vi "TargetUI.vi"() -> ()   [LabVIEW 2019, in "Target.lvclass"]
uses:
  Target.lvclass
  <vilib>/NI/Configuration Framework/Node/NodeRef.ctl
  <vilib>/NI/Configuration Framework/Node/NISE_CEF_Node.lvclass
  <vilib>/NI/AMC/Message Queue.ctl
  <vilib>/NI/AMC/Message.ctl
  <vilib>/NI/Tools/Keyed Array/KeyedArray.ctl
  <vilib>/NI/Configuration Framework/Node/UserEventRef.ctl
  <vilib>/NI/Configuration Framework/Controls/EventCluster.ctl
  C:/Program Files (x86)/National Instruments/LabVIEW 2019/vi.lib/NI/Configuration Framework/Node/NISE_CEF_Node.lvclass
  Target.lvclass/Target.ctl
  Read Source.vi
  Write Source.vi
  <vilib>/NI/AMC/Create Single Message.vi
  <vilib>/NI/AMC/Update Message Routing Info.vi
  <vilib>/NI/AMC/Send Message.vi
  <vilib>/NI/AMC/AMC.lvlib
  Configuration Tool.lvlib
  <vilib>/NI/Tools/Keyed Array/Tools_KeyedArray.lvlib
  <vilib>/NI/Configuration Framework/NISE_CEF_TreeControl.lvlib
panel:
  in  "Main UI Tab":enum32{"Target Information"}(tab)
  in  "Show Documentation":bool
  in  "Host Path to RT Driver VI":path
  in  "Real Time System Destination":string
  in  "user event":T1
  in  "main queue":T2
  in  "node ref":T3
  # "Host Information"
  # "Target Information"
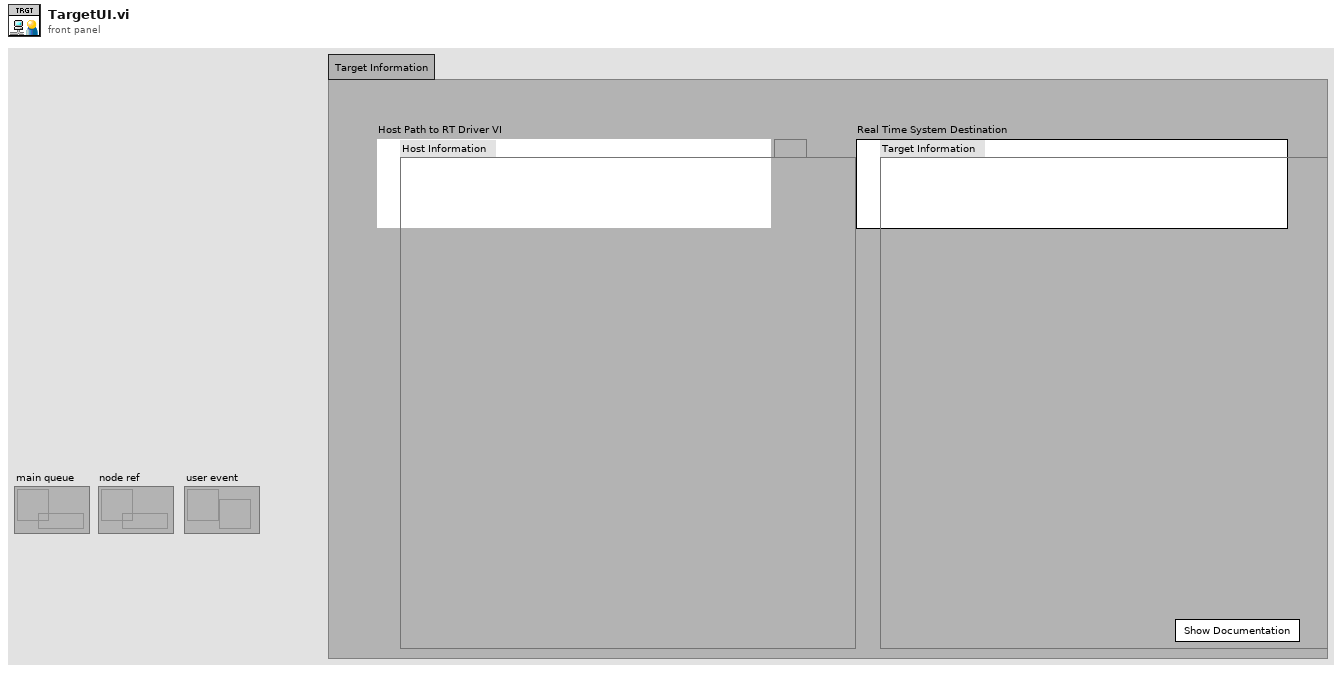
[diagram p1: front panel]
types:
  T1 = typedef "NISE_CEF_Node.lvclass/UserEventRef.ctl" = refnum<user-event>
  T2 = typedef "AMC.lvlib/Message Queue.ctl" = refnum<queue>
  T3 = typedef "NISE_CEF_Node.lvclass/NodeRef.ctl" = refnum<data-value>
  T4 = typedef "VeriStand Custom Device XML Parser.lvlib/Path Cluster.ctl" = cluster{"Path":path, "Path Type":enum16{"Absolute", "To Base", "To Common Doc Dir", "To Application Data Dir"}}
  T5 = typedef "VeriStand Custom Device XML Parser.lvlib/Supported Targets.ctl" = enum16{"All", "Pharlap", "VxWorks", "Windows", "Linux_32_ARM", "Linux_x64", "PharlapWindows", "PharlapVxWorks", "VxWorksWindows"}
  T6 = cluster{"Source":T4, "Real Time System Destination":string, "Supported Target":T5}
  T7 = enum16{"Absolute", "To Base", "To Common Doc Dir", "To Application Data Dir"}
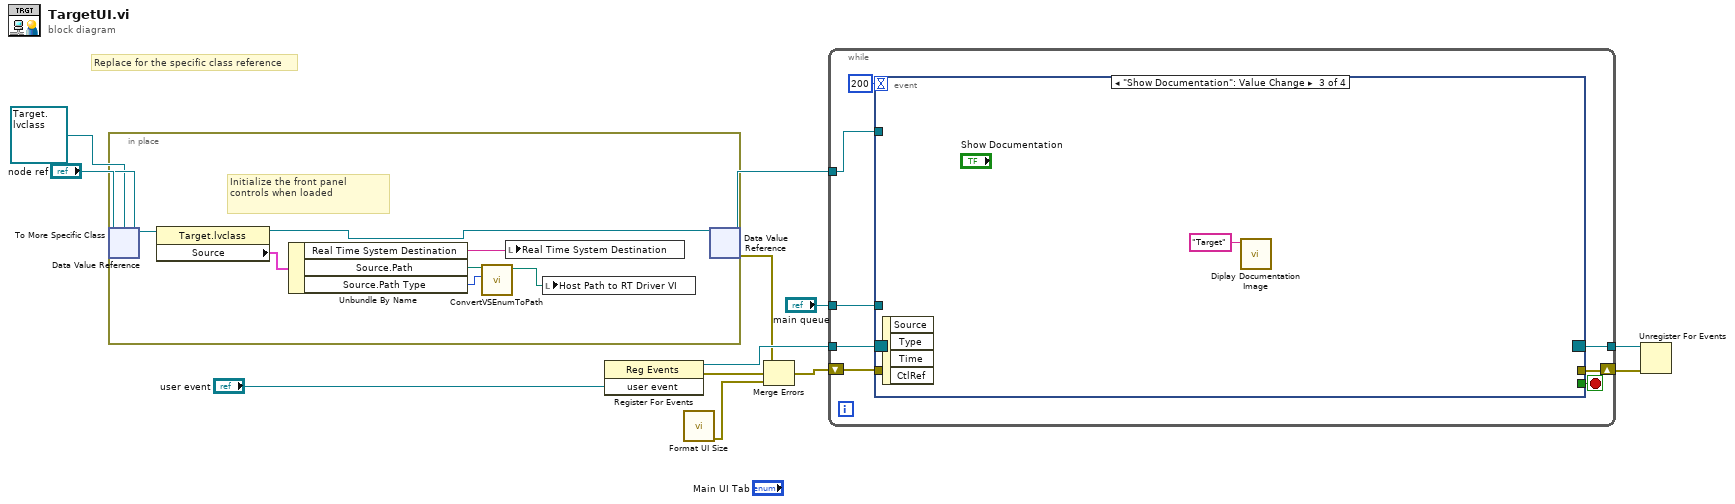
[diagram p0: block diagram]
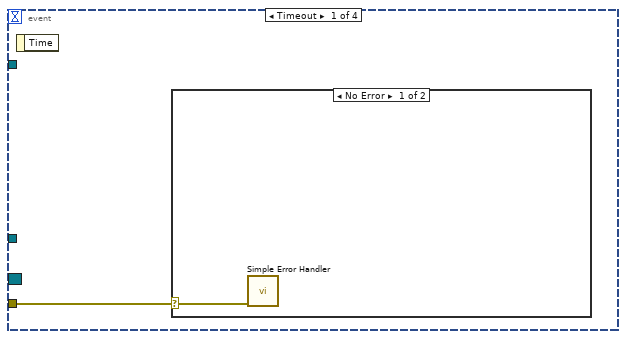
[diagram p2: hidden frame]
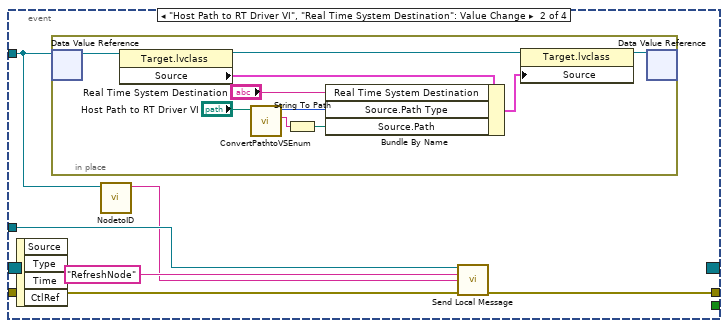
[diagram p4: hidden frame]
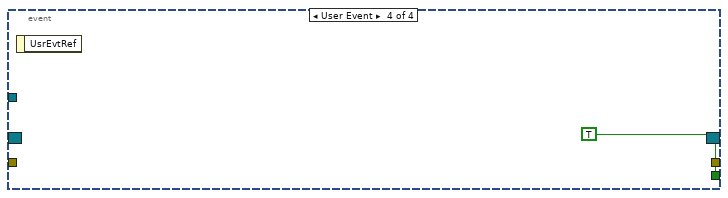
[diagram p5: hidden frame]
diagram:
  # "Replace for the specific class reference"
  n1 = To More Specific Class(target class=refnum<data-value> refnum ("data value reference"), reference="node ref") -> (specific class reference=w6:refnum<data-value>)  [unwired: 1 in, 1 out]
  n2 = in-place {
    # "Initialize the front panel controls when loaded"
    n3 = in-place-dvr #1(w6) -> (w20:refnum<class "Target.lvclass">)  [unwired: 1 out]
    n4 = property class="Target.lvclass"(reference=w20) -> (reference out=w14:refnum<class "Target.lvclass">, "Source"=w15:T6)  [unwired: 1 in, 1 out]
    n5 = Unbundle By Name(w15) -> ("Real Time System Destination"=w17:string, "Source.Path"=w19:path, "Source.Path Type"=w18:T7)
    n6 = call "ConvertVSEnumToPath.vi"("Source.Path Type"=w18, "Path In"=w19) -> ("appended path"=w16:path)  [unwired: 9 in]
    n7 = local write "Real Time System Destination"(w17) -> ()
    n8 = local write "Host Path to RT Driver VI"(w16) -> ()
    n9 = in-place-dvr #1(w14) -> (w13:refnum<data-value>, w3:errorcluster)
  }
  n10 = register-events("user event") -> (reference out=w10:refnum<event-registration>, error out=w4:errorcluster)  [unwired: 2 in]
  n11 = call "Format UI Size.vi"() -> ("error out"=w1:errorcluster)  [unwired: 11 in]
  n12 = Merge Errors(w3, w4, w1) -> (w2:errorcluster)
  n13 = while {
    tunnel: w13 -> [w28]
    tunnel: "main queue" -> [w27]
    tunnel: w10 -> [w25]
    tunnel: [w24] -> w9
    shift-right: [w22] -> w8
    shift-left: w2 -> [w21]
    stop <- w23 stop-if-true
    n14 = event shown="[2] \"Show Documentation\": Value Change" {
      selector: w25 -> [_ _ _ _]
      dyn-events: [_ _ _ _] -> w24
      timeout: 200 -> [_ _ _ _]
      tunnel: w28 -> [_ w34 _ _]
      tunnel: w27 -> [_ w35 _ _]
      tunnel: [_ _ _ TRUE] -> w23
      tunnel: [_ w32 _ _] -> w22
      tunnel: w21 -> [w29 w31 _ _]
      event Timeout {
        n15 = event-data() -> ()  [unwired: 1 in, 1 out]
        n16 = case shown="No Error" w29 {
          selector: w29 -> [w30 _]
          frame No Error {
            n17 = call <vilib>:"Simple Error Handler.vi"("error in (no error)"=w30) -> ()  [unwired: 4 in, 5 out]
          }
          frame Error {
          }
        }
      }
      event "Host Path to RT Driver VI", "Real Time System Destination": Value Change {
        n18 = event-data() -> ()  [unwired: 1 in, 4 out]
        n19 = in-place {
          n20 = in-place-dvr #2(w34) -> (w44:refnum<class "Target.lvclass">)  [unwired: 1 out]
          n21 = property class="Target.lvclass"(reference=w44) -> (reference out=w39:refnum<class "Target.lvclass">, "Source"=w43:T6)  [unwired: 1 in, 1 out]
          n22 = call "ConvertPathtoVSEnum.vi"("Path In"="Host Path to RT Driver VI") -> ("Remaining Path"=w37:string, "VS Enum Out"=w40:T7)  [unwired: 9 in]
          n23 = String To Path(string=w37) -> (path=w38:path)
          n24 = Bundle By Name(cluster=w43, "Real Time System Destination"="Real Time System Destination", "Source.Path Type"=w40, "Source.Path"=w38) -> (w42:T6)
          n25 = property class="Target.lvclass"(reference=w39, "Source"=w42) -> (reference out=w46:refnum<class "Target.lvclass">)  [unwired: 1 in, 1 out]
          n26 = in-place-dvr #2(w46) -> ()  [unwired: 2 out]
        }
        n27 = call <vilib>:"NodetoID.vi"("node ref"=w34) -> ("ID"=w33:string)  [unwired: 9 in, 1 out]
        n28 = call <vilib>:"Send Local Message.vi"("message queue in"=w35, "message name"="RefreshNode" ("Message Name"), "message value"=w33, "error in"=w31) -> ("error out"=w32:errorcluster)  [unwired: 9 in, 2 out]
      }
      event "Show Documentation": Value Change {
        n29 = event-data() -> ()  [unwired: 1 in, 4 out]
        n30 = call "Diplay Documentation Image.vi"("Image Name"="Target") -> ()  [unwired: 10 in, 1 out]
      }
      event User Event {
        n31 = event-data() -> ()  [unwired: 1 in, 1 out]
      }
    }
  }
  n32 = Unregister For Events(event registration refnum=w9, error in=w8) -> ()  [unwired: 1 out]
